vi "insmeas2file.vi"(1 "Numeric":i32, 2 "MeasData":T1, 3 "Array":string[](array[string]), 4 "File Path":path) -> (0 "error out":errorcluster)   [LabVIEW 2010]
panel:
  in  "Case Constant\n(See Context Help)":bool
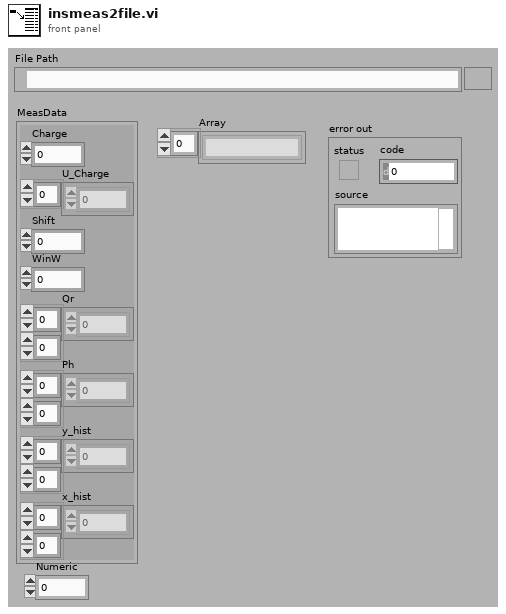
[diagram p1: front panel]
types:
  T1 = cluster{"Charge":i32, "U_Charge":i32[], "Shift":i32, "WinW":i32, "Qr":i32[][], "Ph":i32[][], "y_hist":i32[][], "x_hist":i32[][]}
  T2 = cluster{"Array":string[], "MeasData":cluster{"Charge":i32, "U_Charge":i32[], "Shift":i32, "WinW":i32, "Qr":i32[][], "Ph":i32[][], "y_hist":i32[][], "x_hist":i32[][]}}
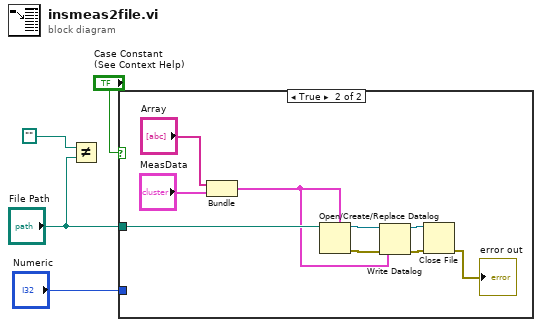
[diagram p0: block diagram]
diagram:
  n1 = Not Equal?(x=path "", y="File Path") -> ()  [unwired: 1 out]
  n2 = case shown="True" "Case Constant\n(See Context Help)" {
    tunnel: "File Path" -> [_ w13]
    tunnel: "Numeric" -> [_ _]
    frame False {
    }
    frame True {
      n3 = Bundle("Array"="Array", "MeasData"="MeasData") -> (w5:T2)  [unwired: 1 in]
      n4 = Open/Create/Replace Datalog(5:w5, 11:w13) -> (0:w11:errorcluster, 3:w10:refnum<k1>)  [unwired: 4 in, 1 out]
      n5 = Write Datalog(4:w11, 6:w5, 7:w10) -> (0:w7:errorcluster, 3:w6:refnum<k1>)
      n6 = Close File(refnum=w6, error in=w7) -> (error out=→"error out":errorcluster)  [unwired: 1 out]
    }
  }
